vi "Hilbert Spectrum.vi"(4 "Waveform":waveform(dbl)) -> (0 "df":dbl, 1 "dt":dbl, 2 "Spectrum":dbl[][](array[numeric]))   [LabVIEW 2013, in "Empirical Mode Decomposition.lvlib"]
uses:
  Empirical Mode Decomposition.lvlib
  <vilib>/Waveform/WDTOps.llb/WDT Waveform Duration DBL.vi
  <vilib>/Analysis/NI_AALPro.lvlib
panel:
  out "Phase":dbl[](graph)
  out "Omega":dbl[](graph)
  out "Frequency":dbl[](graph)
  out "Spectrum":dbl[][](graph)
  out "Waveform Graph":waveform(dbl)[](graph)
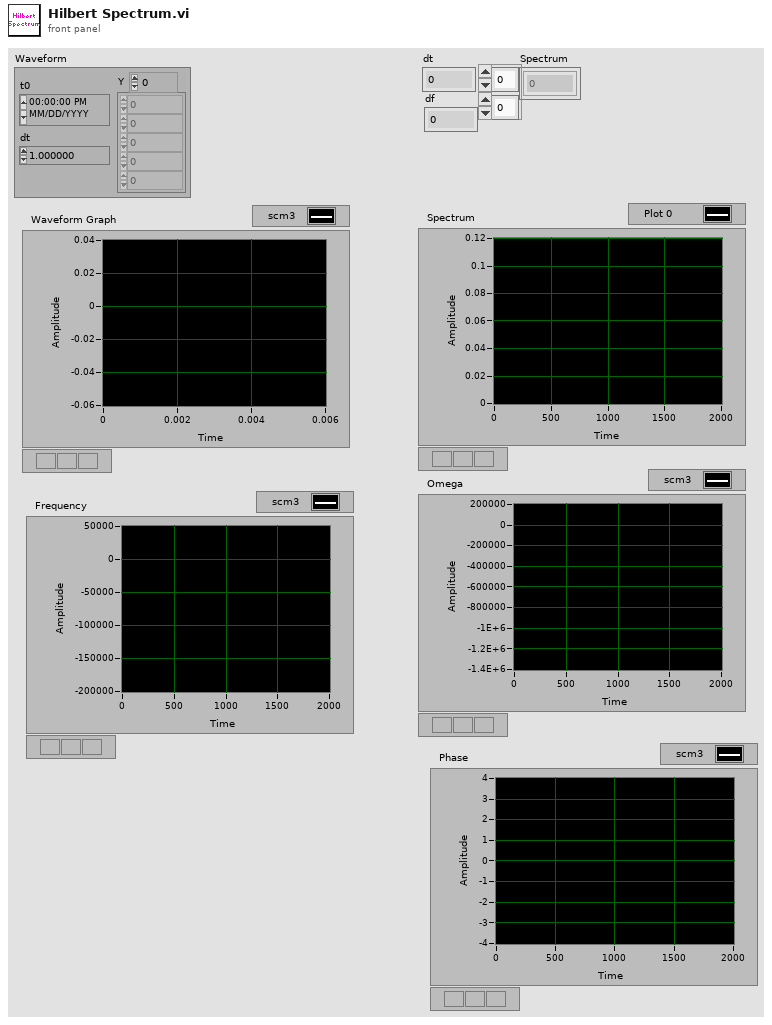
[diagram p1: front panel]
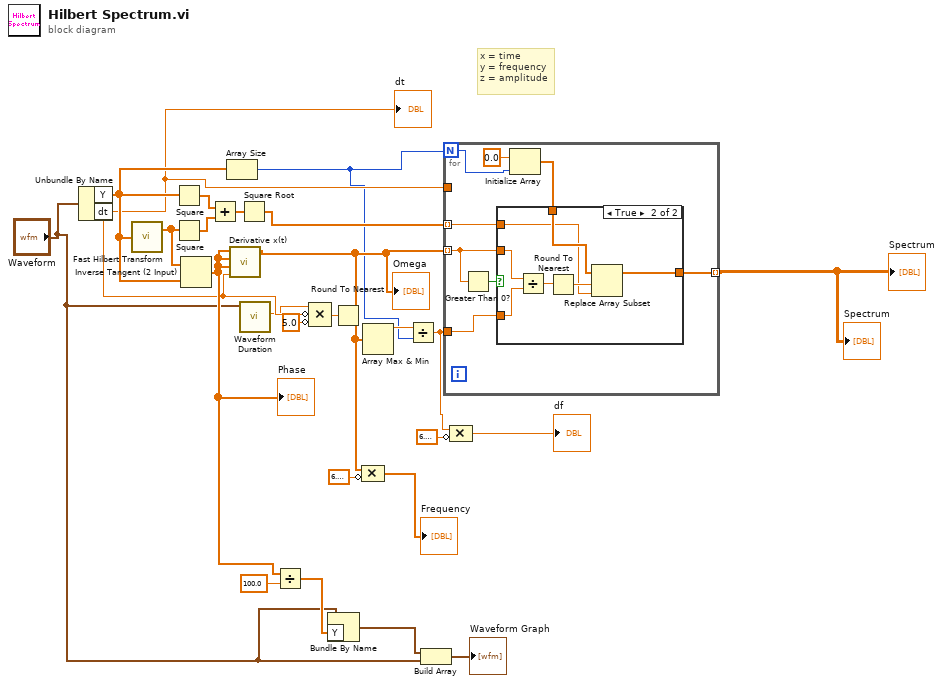
[diagram p0: block diagram]
diagram:
  # "x = time\ny = frequency\nz = amplitude"
  n1 = Unbundle By Name("Waveform") -> ("Y"=w20:dbl[], "dt"=w5:dbl)
  "dt" <- w5
  n2 = call <vilib>:"Fast Hilbert Transform.vi"("X"=w20) -> ("Hilbert{X}"=w19:dbl[])  [unwired: 1 out]
  n3 = Square(x=w20) -> (x^2=w18:dbl[])
  n4 = Square(x=w19) -> (x^2=w17:dbl[])
  n5 = Inverse Tangent (2 Input)(1:w20, 2:w19) -> (0:w8:dbl[])
  "Phase" <- w8
  n6 = Add(x=w18, y=w17) -> (x+y=w16:dbl[])
  n7 = Array Size(array=w20) -> (size(s)=w1:i32)
  n8 = call <vilib>:"Derivative x(t).vi"("dt"=w5, "Final Condition"=w8, "Initial Condition"=w8, "X"=w8) -> ("dX/dt"=w7:dbl[])  [unwired: 6 in, 1 out]
  "Omega" <- w7
  n9 = Square Root(x=w16) -> (sqrt(x)=w15:dbl[])
  n10 = call-poly <vilib>:"Waveform Duration.vi"("waveform in"="Waveform") -> ("duration"=w2:dbl)  [unwired: 8 in, 2 out]
  n11 = Divide(x=w8, y=100.0 ("value")) -> (x/y=w21:dbl[])
  n12 = Compound Arithmetic op=MULTIPLY(w2, invert w5, invert 5.0 ("value")) -> (w3:dbl)
  n13 = Bundle By Name(cluster="Waveform", "Y"=w21) -> (w23:waveform(dbl))
  n14 = Round To Nearest(number=w3) -> ()  [unwired: 1 out]
  n15 = Compound Arithmetic op=MULTIPLY(w7, invert 6.283185307179586) -> (→"Frequency":dbl[])
  n16 = Array Max & Min(array=w7) -> (max value=w25:dbl)  [unwired: 3 out]
  n17 = Divide(x=w25, y=w1) -> (x/y=w9:dbl)
  n18 = Build Array(w23, "Waveform") -> (→"Waveform Graph":waveform(dbl)[])
  n19 = for {
    N: w1 -> [w29]
    tunnel: w5 -> [_]
    tunnel: w15 -> [w27] mode=indexing
    tunnel: w7 -> [w32] mode=indexing
    tunnel: w9 -> [w31]
    tunnel: [w26] -> w14 mode=indexing
    n20 = Greater Than 0?(x=w32) -> (x > 0?=w33:bool)
    n21 = Initialize Array(0.0 ("element"), w29) -> (w28:dbl[])
    n22 = case shown="True" w33 {
      tunnel: w32 -> [_ w41]
      tunnel: w31 -> [_ w40]
      tunnel: w28 -> [w34 w37]
      tunnel: w27 -> [_ w36]
      tunnel: [w34 w35] -> w26
      frame False {
      }
      frame True {
        n23 = Divide(x=w41, y=w40) -> (x/y=w39:dbl)
        n24 = Round To Nearest(number=w39) -> (nearest integer value=w38:dbl)
        n25 = Replace Array Subset(array=w37, new element=w36, index=w38) -> (w35:dbl[])
      }
    }
  }
  "Spectrum" <- w14
  "Spectrum" <- w14
  n26 = Compound Arithmetic op=MULTIPLY(w9, invert 6.283185307179586) -> (→"df":dbl)
